vi "SeCrTs-Data Transfer Loop RD.vi"(9 "Message Queue 2":refnum<queue>, 11 "Data FIFO Ref":T1) -> ()   [LabVIEW 2022 SP3]
uses:
  RT Controls/SeCrTs-Message Cluster_R.ctl
  RT Controls/SeCrTs-Data FIFO.ctl
  RT Controls/SeCrTs-DiplayPC comm ctrl.ctl
  <vilib>/Platform/TimedLoop/XDataNode/timing_clust.ctl
  <vilib>/Platform/TimedLoop/XDataNode/nitl_modes.ctl
  <vilib>/Platform/TimedLoop/XDataNode/wakeup.ctl
  RT Controls/SeCrTs-RD Data transfer data type.ctl
  RT Support/SeCrTs-RT_Global_R.vi
  <vilib>/platform/TimedLoop/XDataNode/XDataNode.xnode
  <resource>/objmgr/ni.dex.rc
  <vilib>/Platform/TimedLoop/XDataNode/XDNodeRunTimeDep.lvlib
panel:
  out "Total Elements Written":u64
  out "x-y":u32
  in  "Message Queue":refnum<queue>
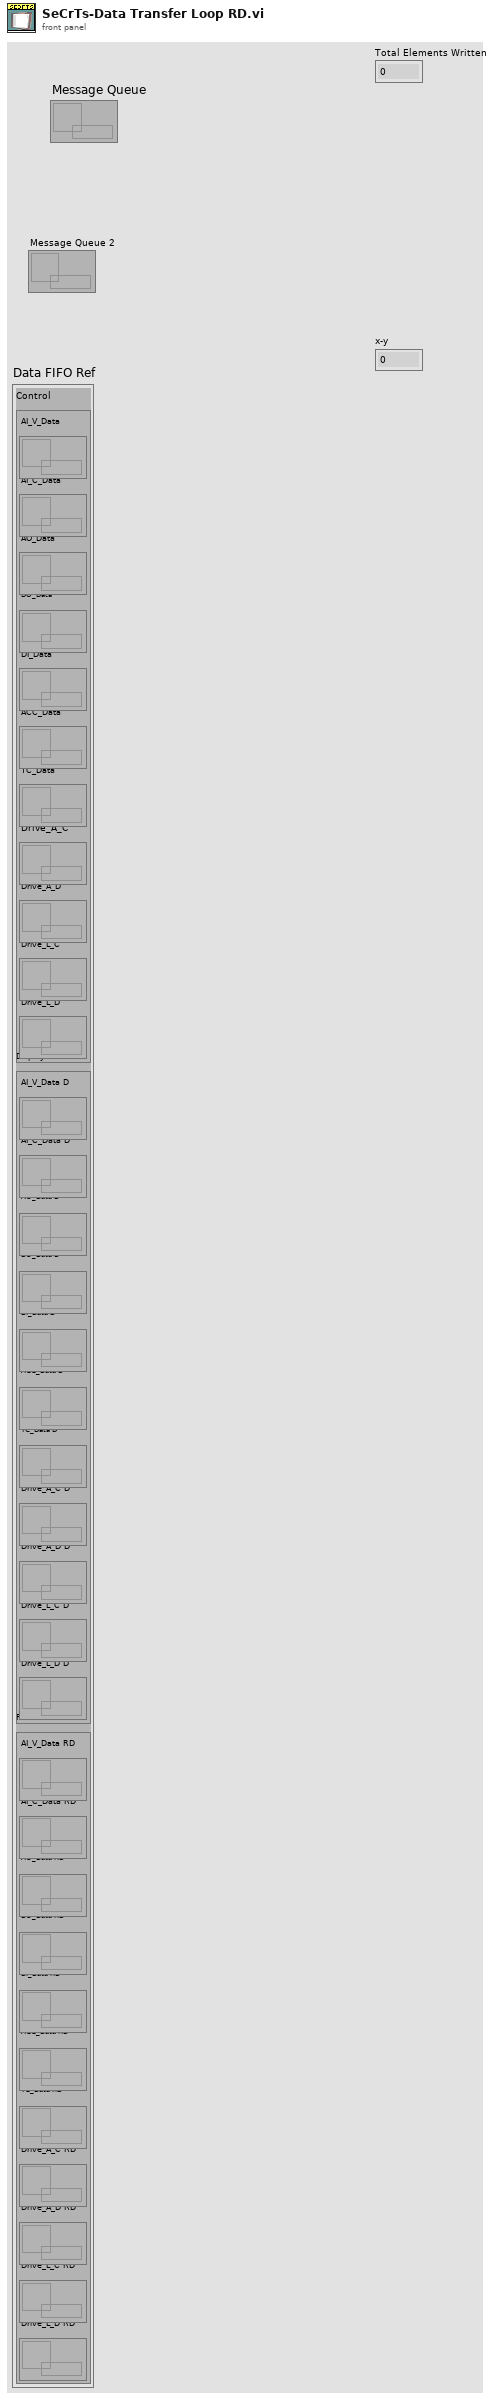
[diagram p1: front panel]
types:
  T1 = typedef "SeCrTs-Data FIFO.ctl" = cluster{"Control":cluster{"AI_V_Data":refnum<queue>, "AI_C_Data":refnum<queue>, "AO_Data":refnum<queue>, "DO_Data":refnum<queue>, "DI_Data":refnum<queue>, "ACC_Data":refnum<queue>, "TC_Data":refnum<queue>, "Drive_A_C":refnum<queue>, "Drive_A_D":refnum<queue>, "Drive_L_C":refnum<queue>, "Drive_L_D":refnum<queue>}, "Display":cluster{"AI_V_Data D":refnum<queue>, "AI_C_Data D":refnum<queue>, "AO_Data D":refnum<queue>, "DO_Data D":refnum<queue>, "DI_Data D":refnum<queue>, "ACC_Data D":refnum<queue>, "TC_Data D":refnum<queue>, "Drive_A_C D":refnum<queue>, "Drive_A_D D":refnum<queue>, "Drive_L_C D":refnum<queue>, "Drive_L_D D":refnum<queue>}, "RD":cluster{"AI_V_Data RD":refnum<queue>, "AI_C_Data RD":refnum<queue>, "AO_Data RD":refnum<queue>, "DO_Data RD":refnum<queue>, "DI_Data RD":refnum<queue>, "ACC_Data RD":refnum<queue>, "TC_Data RD":refnum<queue>, "Drive_A_C RD":refnum<queue>, "Drive_A_D RD":refnum<queue>, "Drive_L_C RD":refnum<queue>, "Drive_L_D RD":refnum<queue>}}
  T2 = typedef "SeCrTs-DiplayPC comm ctrl.ctl" = enum16{"Initialize", "Listen for UI Writer", "Send RT Data"}
  T3 = typedef "XDNodeRunTimeDep.lvlib/timing_clust.ctl" = cluster{"Expected End [f-1]":u64, "Actual End [f-1]":u64, "Finished Late? [f-1]":bool, "Expected End [i-1]":u64, "Actual End [i-1]":u64, "Finished Late? [i-1]":bool, "Expected Start [i]":u64, "Actual Start [i]":u64, "Expected Start [f]":u64, "Actual Start [f]":u64, "Source Name":string, "Structure Name":string, "Period":i64, "Deadline":i64, "Offset":i64, "Start":i64, "Priority":i32, "Timeout":i32, "Mode":T4, "Wakeup Reason":T5, "Error":errorcluster, "Source Type":string, "Secondary Source Type":string, "Global End Time":u64, "Global Start Time":u64, "Frame Duration":u64, "Iteration Duration":u64, "Assigned CPU":i32, "I/O Scan Engine Mode":u32}
  T4 = typedef "XDNodeRunTimeDep.lvlib/nitl_modes.ctl" = enum32{"No Change", "Process missed periods, maintain original phase", "Discard missed periods, maintain original phase", "Process missed periods, ignore original phase", "Discard missed periods, ignore original phase"}
  T5 = typedef "XDNodeRunTimeDep.lvlib/wakeup.ctl" = enum32{"Normal", "Aborted", "Asynchronous wakeup", "Timing source error", "Timed loop error", "Timeout"}
  T6 = typedef "SeCrTs-RD Data transfer data type.ctl" = cluster{"AI_V_Data":waveform(dbl)[][], "AI_C_Data":waveform(dbl)[][], "AO_Data":waveform(dbl)[][], "DO_Data":waveform(dbl)[][], "DI_Data":digitalwaveform[][], "ACC_Data":waveform(dbl)[][], "TC Data":waveform(dbl)[][], "Drive_A_C":waveform(dbl)[][], "Drive_A_D":waveform(dbl)[][], "Drive_L_C":waveform(dbl)[][], "Drive_L_D":waveform(dbl)[][]}
  T7 = cluster{"Start DAQ":bool, "Stop DAQ":bool, "RT Stop":bool, "RT Exit":bool, "Start Seq":bool}
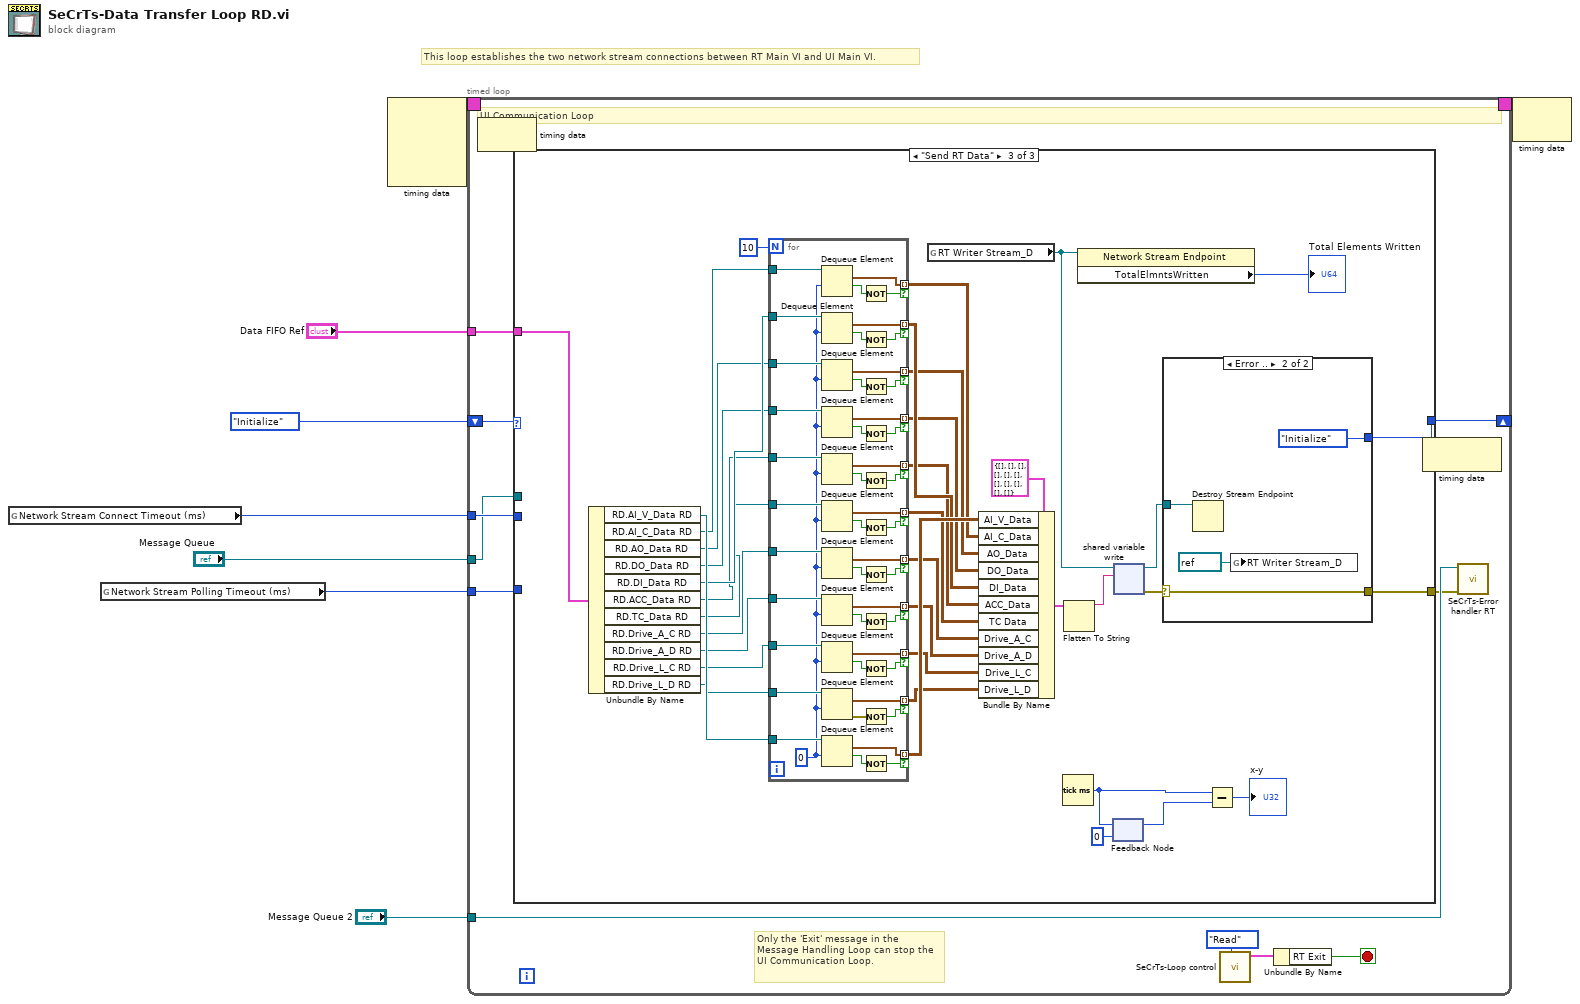
[diagram p0: block diagram]
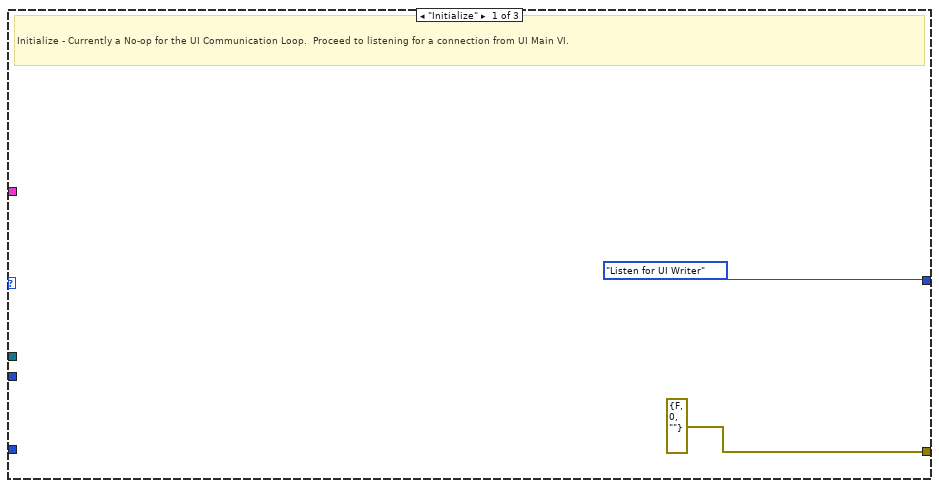
[diagram p2: hidden frame]
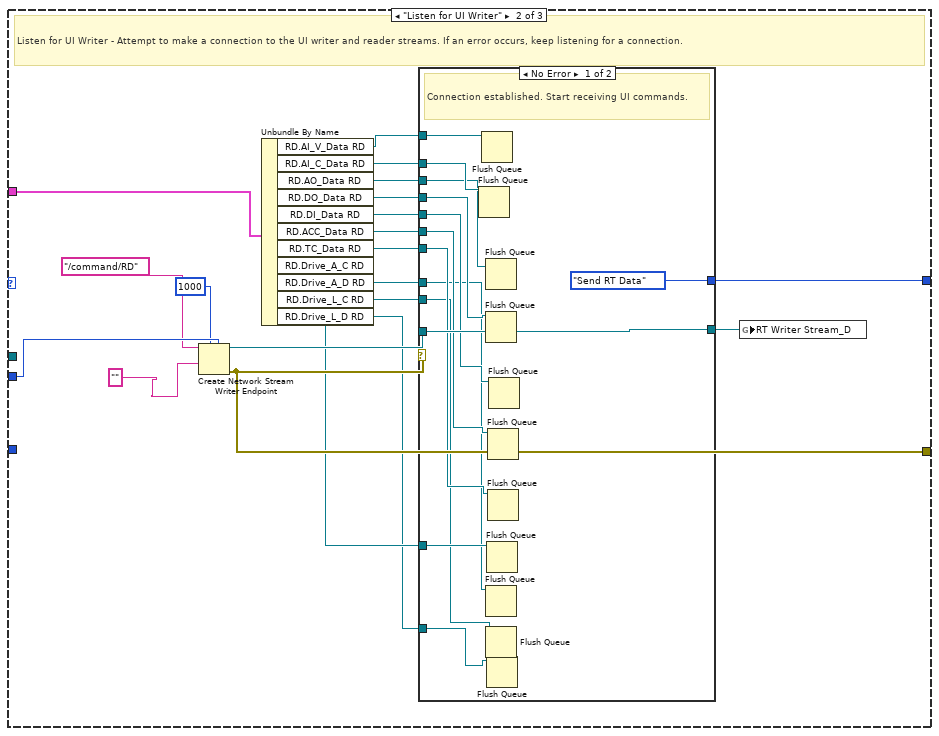
[diagram p3: hidden frame]
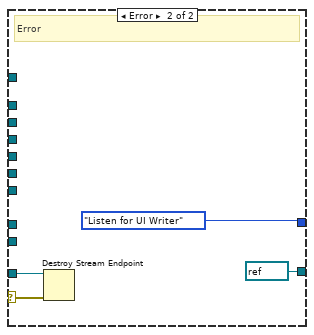
[diagram p4: hidden frame]
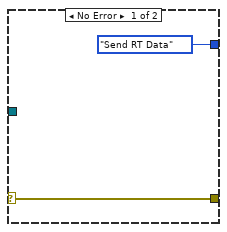
[diagram p5: hidden frame]
diagram:
  # "This loop establishes the two network stream connections between RT Main VI and UI Main VI."
  n1 = global read "SeCrTs-RT_Global_R.vi" "Network Stream Connect Timeout (ms)"() -> (w6:i32)
  n2 = global read "SeCrTs-RT_Global_R.vi" "Network Stream Polling Timeout (ms)"() -> (w7:i32)
  n3 = node-c288() -> (w2:T3)  [unwired: 4 in]
  n4 = timed-loop {
    tunnel: "Message Queue" -> [w16]
    tunnel: w7 -> [w19]
    tunnel: w6 -> [w18]
    shift-right: [w17] -> _
    shift-left: SeCrTs-DiplayPC_comm_ctrl."Initialize" -> [w15]
    tunnel: "Data FIFO Ref" -> [w14]
    tunnel: "Message Queue 2" -> [w10]
    timing: w2 -> [_]
    timing-out: [_] -> w1
    stop <- w11 stop-if-true
    # "Only the 'Exit' message in the  Message Handling Loop can stop the UI Communication Loop."
    # "UI Communication Loop"
    n5 = node-c288() -> ()  [unwired: 1 in, 1 out]
    n6 = case shown="\"Send RT Data\"" w15 {
      tunnel: [errorcluster {"status"=FALSE, "code"=0, "source"=""} ("error IO") w42 w96] -> w9
      tunnel: w18 -> [_ w41 _]
      tunnel: w16 -> [_ _ _]
      tunnel: w19 -> [_ _ _]
      tunnel: [SeCrTs-DiplayPC_comm_ctrl."Listen for UI Writer" w40 w94] -> w17
      tunnel: w14 -> [_ w37 w89]
      frame "Initialize" {
        # "Initialize - Currently a No-op for the UI Communication Loop.  Proceed to listening for a connection from UI Main VI."
      }
      frame "Listen for UI Writer" {
        # "Listen for UI Writer - Attempt to make a connection to the UI writer and reader streams. If an error occurs, keep listening for a connection."
        n7 = Create Network Stream Writer Endpoint(5:w41, 7:1000 ("writer buffer size"), 9:"" ("reader url"), 11:"/command/RD" ("reader url")) -> (0:w42:errorcluster, 3:w43:refnum<k21>)  [unwired: 3 in]
        n8 = Unbundle By Name(w37) -> ("RD.AI_V_Data RD"=w36:refnum<queue>, "RD.AI_C_Data RD"=w35:refnum<queue>, "RD.AO_Data RD"=w34:refnum<queue>, "RD.DO_Data RD"=w33:refnum<queue>, "RD.DI_Data RD"=w32:refnum<queue>, "RD.ACC_Data RD"=w31:refnum<queue>, "RD.TC_Data RD"=w30:refnum<queue>, "RD.Drive_A_C RD"=w29:refnum<queue>, "RD.Drive_A_D RD"=w28:refnum<queue>, "RD.Drive_L_C RD"=w27:refnum<queue>, "RD.Drive_L_D RD"=w26:refnum<queue>)
        n9 = case shown="No Error" w42 {
          selector: w42 -> [_ w58]
          tunnel: w43 -> [w55 w60]
          tunnel: [SeCrTs-DiplayPC_comm_ctrl."Send RT Data" SeCrTs-DiplayPC_comm_ctrl."Listen for UI Writer"] -> w40
          tunnel: [w55 refnum<k21> refnum ("reader url")] -> w24
          tunnel: w36 -> [w54 _]
          tunnel: w35 -> [w53 _]
          tunnel: w34 -> [w52 _]
          tunnel: w33 -> [w51 _]
          tunnel: w32 -> [w50 _]
          tunnel: w31 -> [w49 _]
          tunnel: w30 -> [w48 _]
          tunnel: w29 -> [w47 _]
          tunnel: w28 -> [w46 _]
          tunnel: w27 -> [w45 _]
          tunnel: w26 -> [w44 _]
          frame No Error {
            # "Connection established. Start receiving UI commands."
            n10 = Flush Queue(queue=w53) -> ()  [unwired: 1 in, 3 out]
            n11 = Flush Queue(queue=w54) -> ()  [unwired: 1 in, 3 out]
            n12 = Flush Queue(queue=w52) -> ()  [unwired: 1 in, 3 out]
            n13 = Flush Queue(queue=w51) -> ()  [unwired: 1 in, 3 out]
            n14 = Flush Queue(queue=w46) -> ()  [unwired: 1 in, 3 out]
            n15 = Flush Queue(queue=w45) -> ()  [unwired: 1 in, 3 out]
            n16 = Flush Queue(queue=w47) -> ()  [unwired: 1 in, 3 out]
            n17 = Flush Queue(queue=w44) -> ()  [unwired: 1 in, 3 out]
            n18 = Flush Queue(queue=w49) -> ()  [unwired: 1 in, 3 out]
            n19 = Flush Queue(queue=w48) -> ()  [unwired: 1 in, 3 out]
            n20 = Flush Queue(queue=w50) -> ()  [unwired: 1 in, 3 out]
          }
          frame Error {
            # "Error"
            n21 = Destroy Stream Endpoint(8:w58, 11:w60) -> ()  [unwired: 1 out]
          }
        }
        n22 = global write "SeCrTs-RT_Global_R.vi" "RT Writer Stream_D"(w24) -> ()
      }
      frame "Send RT Data" {
        n23 = Unbundle By Name(w89) -> ("RD.AI_V_Data RD"=w90:refnum<queue>, "RD.AI_C_Data RD"=w82:refnum<queue>, "RD.AO_Data RD"=w78:refnum<queue>, "RD.DO_Data RD"=w76:refnum<queue>, "RD.DI_Data RD"=w79:refnum<queue>, "RD.ACC_Data RD"=w74:refnum<queue>, "RD.TC_Data RD"=w72:refnum<queue>, "RD.Drive_A_C RD"=w70:refnum<queue>, "RD.Drive_A_D RD"=w68:refnum<queue>, "RD.Drive_L_C RD"=w66:refnum<queue>, "RD.Drive_L_D RD"=w64:refnum<queue>)
        n24 = for {
          N: 10 -> [_]
          tunnel: w90 -> [w142]
          tunnel: [w141] -> w86 mode=indexing if=w139
          tunnel: w82 -> [w138]
          tunnel: [w137] -> w81 mode=indexing if=w133
          tunnel: w79 -> [w136]
          tunnel: [w135] -> w80 mode=indexing if=w131
          tunnel: w78 -> [w130]
          tunnel: [w129] -> w77 mode=indexing if=w112
          tunnel: w76 -> [w128]
          tunnel: [w127] -> w75 mode=indexing if=w98
          tunnel: w74 -> [w126]
          tunnel: [w125] -> w73 mode=indexing if=w101
          tunnel: w72 -> [w124]
          tunnel: [w123] -> w71 mode=indexing if=w103
          tunnel: w70 -> [w122]
          tunnel: [w121] -> w69 mode=indexing if=w104
          tunnel: w68 -> [w120]
          tunnel: [w119] -> w67 mode=indexing if=w105
          tunnel: w66 -> [w118]
          tunnel: [w117] -> w65 mode=indexing if=w107
          tunnel: w64 -> [w116]
          tunnel: [w115] -> w63 mode=indexing if=w108
          w114 = 0 ("timeout in ms (-1)")
          n25 = Dequeue Element(queue=w138, timeout in ms (-1)=w114) -> (element=w137:waveform(dbl)[], timed out?=w134:bool)  [unwired: 1 in, 2 out]
          n26 = Dequeue Element(queue=w136, timeout in ms (-1)=w114) -> (element=w135:digitalwaveform[], timed out?=w132:bool)  [unwired: 1 in, 2 out]
          n27 = Dequeue Element(queue=w130, timeout in ms (-1)=w114) -> (element=w129:waveform(dbl)[], timed out?=w113:bool)  [unwired: 1 in, 2 out]
          n28 = Dequeue Element(queue=w128, timeout in ms (-1)=w114) -> (element=w127:waveform(dbl)[], timed out?=w99:bool)  [unwired: 1 in, 2 out]
          n29 = Dequeue Element(queue=w126, timeout in ms (-1)=w114) -> (element=w125:waveform(dbl)[], timed out?=w100:bool)  [unwired: 1 in, 2 out]
          n30 = Dequeue Element(queue=w124, timeout in ms (-1)=w114) -> (element=w123:waveform(dbl)[], timed out?=w102:bool)  [unwired: 1 in, 2 out]
          n31 = Dequeue Element(queue=w122, timeout in ms (-1)=w114) -> (element=w121:waveform(dbl)[], timed out?=w111:bool)  [unwired: 1 in, 2 out]
          n32 = Dequeue Element(queue=w120, timeout in ms (-1)=w114) -> (element=w119:waveform(dbl)[], timed out?=w106:bool)  [unwired: 1 in, 2 out]
          n33 = Dequeue Element(queue=w118, timeout in ms (-1)=w114) -> (element=w117:waveform(dbl)[], timed out?=w110:bool)  [unwired: 1 in, 2 out]
          n34 = Dequeue Element(queue=w116, timeout in ms (-1)=w114) -> (element=w115:waveform(dbl)[], error out=w109:errorcluster)  [unwired: 1 in, 2 out]
          n35 = Dequeue Element(queue=w142, timeout in ms (-1)=w114) -> (element=w141:waveform(dbl)[], timed out?=w140:bool)  [unwired: 1 in, 2 out]
          n36 = Not(x=w134) -> (.not. x?=w133:bool)
          n37 = Not(x=w132) -> (.not. x?=w131:bool)
          n38 = Not(x=w113) -> (.not. x?=w112:bool)
          n39 = Not(x=w99) -> (.not. x?=w98:bool)
          n40 = Not(x=w100) -> (.not. x?=w101:bool)
          n41 = Not(x=w102) -> (.not. x?=w103:bool)
          n42 = Not(x=w111) -> (.not. x?=w104:bool)
          n43 = Not(x=w106) -> (.not. x?=w105:bool)
          n44 = Not(x=w110) -> (.not. x?=w107:bool)
          n45 = Not(x=w109) -> (.not. x?=w108:bool)
          n46 = Not(x=w140) -> (.not. x?=w139:bool)
        }
        n47 = global read "SeCrTs-RT_Global_R.vi" "RT Writer Stream_D"() -> (w85:refnum<k21>)
        n48 = Bundle By Name(cluster=T6 {"AI_V_Data"=[], "AI_C_Data"=[], "AO_Data"=[], "DO_Data"=[], "DI_Data"=[], "ACC_Data"=[], "TC Data"=[], "Drive_A_C"=[], "Drive_A_D"=[], "Drive_L_C"=[], "Drive_L_D"=[]} ("Cluster"), "AI_V_Data"=w86, "AI_C_Data"=w81, "AO_Data"=w77, "DO_Data"=w75, "DI_Data"=w80, "ACC_Data"=w73, "TC Data"=w71, "Drive_A_C"=w69, "Drive_A_D"=w67, "Drive_L_C"=w65, "Drive_L_D"=w63) -> (w62:T6)
        n49 = Tick Count (ms)() -> (millisecond timer value=w93:u32)
        n50 = Flatten To String(anything=w62) -> (data string=w61:string)  [unwired: 3 in, 2 out]
        n51 = property class="Network Stream Endpoint"(reference=w85) -> ("TotalElmntsWritten"=→"Total Elements Written":u64)  [unwired: 1 in, 2 out]
        n52 = feedback-in #1(w93) -> ()
        n53 = feedback #1(u32 0 ("millisecond timer value")) -> (w92:u32)
        n54 = shared-variable-write(w85, w61) -> (w95:refnum<k21>, w97:errorcluster)  [unwired: 2 in, 1 out]
        n55 = case shown="Error .." w97 {
          selector: w97 -> [w144 w145]
          tunnel: [w144 w145] -> w96
          tunnel: w95 -> [_ w148]
          tunnel: [SeCrTs-DiplayPC_comm_ctrl."Send RT Data" SeCrTs-DiplayPC_comm_ctrl."Initialize"] -> w94
          frame No Error {
          }
          frame Error {
            n56 = Destroy Stream Endpoint(11:w148) -> ()  [unwired: 1 in, 1 out]
            n57 = global write "SeCrTs-RT_Global_R.vi" "RT Writer Stream_D"(refnum<k21> refnum ("RT Writer Stream_D")) -> ()
          }
        }
        n58 = Subtract(x=w93, y=w92) -> (x-y=→"x-y":u32)
      }
    }
    n59 = call "SeCrTs-Loop control.vi"("Action"=enum16{"Init", "Write", "Read"}."Read") -> ("Loop Control out"=w13:T7)  [unwired: 9 in, 1 out]
    n60 = Unbundle By Name(w13) -> ("RT Exit"=w11:bool)
    n61 = node-c288() -> ()  [unwired: 1 in, 1 out]
    n62 = call "SeCrTs-Error handler RT.vi"("error in"=w9, "Message Queue"=w10) -> ()  [unwired: 8 in, 2 out]
  }
  n63 = node-c288(w1) -> ()  [unwired: 1 out]
